vi "OpenCVCam_Init.vi"(8 "ErrorIn":errorcluster, 10 "CmdData":variant, 11 "OpenCVCamIn":refnum<class>) -> (0 "ErrorOut":errorcluster, 2 "ReplyData":variant, 3 "OpenCVCamOut":refnum<class>, 4 "Exit":bool)   [LabVIEW 2021, in "OpenCVCam.lvclass"]
uses:
  OpenCVCam.lvclass
  OpenCVCam.lvclass/OpenCVCam.ctl
  State.ctl
  C:/Localdata/Projects/TriekselSoft/TriekselsoftApplicationFramework/Source/.Externals/Library_EmguCV/Emgu.CV.Platform.NetStandard.dll
  .Externals/Library_EmguCV/Emgu.CV.Platform.NetStandard.dll
  C:/Localdata/Projects/TriekselSoft/TriekselsoftApplicationFramework/Source/.Externals/Library_YAF/YAFTAF/YAFTAF.lvclass
  C:/Localdata/Projects/TriekselSoft/TriekselsoftApplicationFramework/Source/.Externals/Library_YAF/YActor/YActor.lvclass
  C:/Localdata/Projects/TriekselSoft/TriekselsoftApplicationFramework/Source/.Externals/Interface_UserInterface_IFrontPanel/IFrontPanel/IFrontPanel.lvclass
  C:/Localdata/Projects/TriekselSoft/TriekselsoftApplicationFramework/Source/IInterface/IInterface.lvclass
  C:/Localdata/Projects/TriekselSoft/TriekselsoftApplicationFramework/Source/.Externals/Interface_Object_ICreateDestroy/ICreateDestroy/ICreateDestroy.lvclass
  C:/Localdata/Projects/TriekselSoft/TriekselsoftApplicationFramework/Source/.Externals/Interface_Object_IPersistentData/IPersistentData/IPersistentData.lvclass
  C:/Localdata/Projects/TriekselSoft/TriekselsoftApplicationFramework/Source/.Externals/Interface_TAF_ITAFObject/ITAFObject/ITAFObject.lvclass
  C:/Localdata/Projects/TriekselSoft/TriekselsoftApplicationFramework/Source/YAFTAFObjects/OpenCVCam/OpenCVCam.lvclass
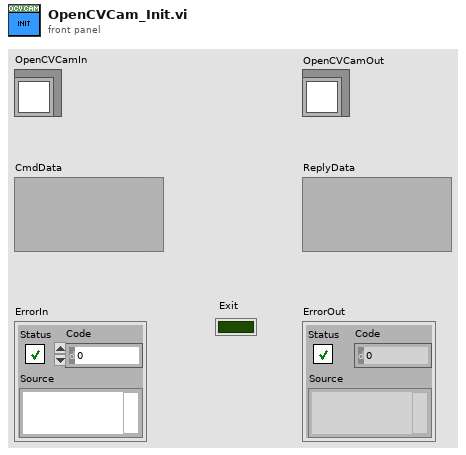
[diagram p1: front panel]
types:
  T1 = typedef "OpenCVCam.lvclass/State.ctl" = enum16{"Idle", "Initialized", "Acquiring"}
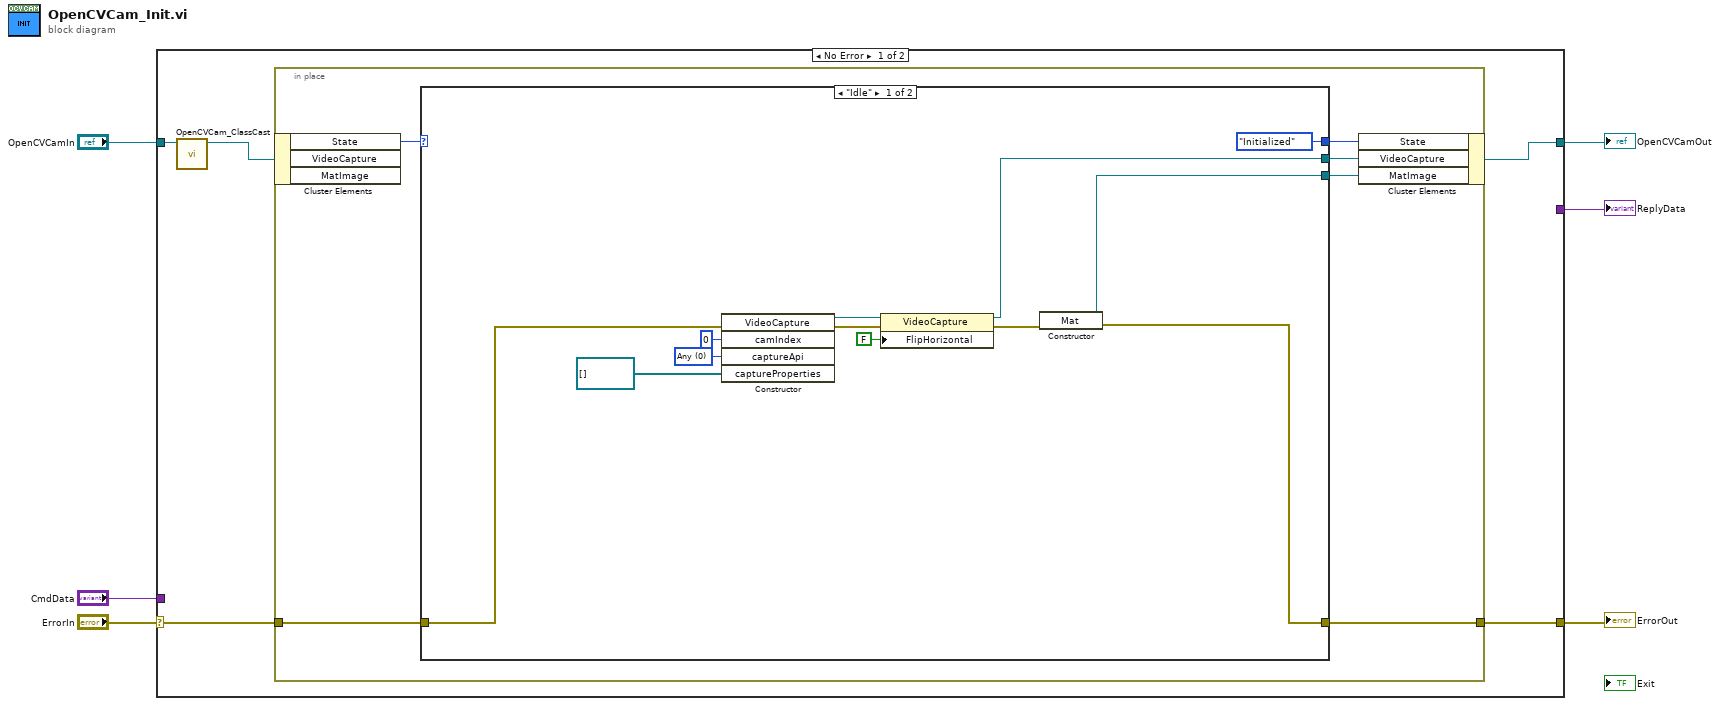
[diagram p0: block diagram]
diagram:
  n1 = case shown="No Error" "ErrorIn" {
    selector: "ErrorIn" -> [w11 w34]
    tunnel: [w10 w34] -> w5
    tunnel: [_ w33] -> w3
    tunnel: "CmdData" -> [_ w33]
    tunnel: "OpenCVCamIn" -> [w9 w32]
    tunnel: [w7 w32] -> w1
    frame No Error {
      n2 = call "OpenCVCam_ClassCast.vi"("OpenCVCamIn"=w9) -> ("OpenCVCamOut"=w8:refnum<class "OpenCVCam.lvclass">)  [unwired: 10 in]
      n3 = in-place {
        in-place-border: w11 -> [w17]
        in-place-border: [w16] -> w10
        n4 = in-place-cluster #1(w8) -> ("State"=w15:T1)  [unwired: 2 out]
        n5 = case shown="\"Idle\"" w15 {
          selector: w15 -> [_ w30]
          tunnel: [w27 w31] -> w16
          tunnel: w17 -> [w29 w31]
          tunnel: [State."Initialized" ("State") w30] -> w14
          tunnel: [w19 _] -> w13
          tunnel: [w21 _] -> w12
          frame "Idle" {
            w24 = 0 items=["Any"=0, "Vfw, V4L, V4L2"=200, "Firewire, IEEE1394, DC1394, CMU1394"=300, "QT"=500, "Unicap"=600, "DShow"=700, "Pvapi"=800, "OpenNI"=900, "OpenNIAsus"=910, "Android"=1000, "XiApi"=1100, "AVFoundation"=1200, "Giganetix"=1300, "Msmf"=1400, "Winrt"=1410, "IntelPerc"=1500, "Openni2"=1600, "Openni2Asus"=1610, "Gphoto2"=1700, "Gstreamer"=1800, "Ffmpeg"=1900, "Images"=2000, "Aravis"=2100, "OpencvMjpeg"=2200, "IntelMfx"=2300, "Xine"=2400] ("captureApi")
            n6 = constructor class="VideoCapture"(error in=w29, "camIndex"=0, "captureApi"=w24, "captureProperties"=refnum<k24>[] []) -> (reference out=w20:refnum<k24>, error out=w28:errorcluster)  [unwired: 2 in, 4 out]
            n7 = property class="VideoCapture"(reference=w20, error in=w28, "FlipHorizontal"=FALSE) -> (reference out=w19:refnum<k24>, error out=w26:errorcluster)
            n8 = constructor class="Mat"(error in=w26) -> (reference out=w21:refnum<k24>, error out=w27:errorcluster)  [unwired: 2 in, 1 out]
          }
          frame "Initialized", "Acquiring" {
          }
        }
        n9 = in-place-cluster #1("State"=w14, "VideoCapture"=w13, "MatImage"=w12) -> (w7:refnum<class "OpenCVCam.lvclass">)
      }
    }
    frame Error {
    }
  }
  "ErrorOut" <- w5
  "OpenCVCamOut" <- w1
  "ReplyData" <- w3
